vi "PID (Parallel) with monitoring.vi"(7 "Error":dbl, 12 "Proportional Gain":dbl=1.0, 13 "Integral Gain":dbl=1.0, 14 "Derivative Gain":dbl=1.0, 15 "High Frequency [s] (Tf)":dbl=1.0) -> (6 "Separate output":dbl[](array[numeric]), 8 "Output":dbl)   [LabVIEW 2017]
doc: "Constructs a PID model in transfer function form."
uses:
  <vilib>/Simulation/Model Libraries/PID/subVIs/SIM PID Derivative Gain.vi
  <vilib>/Simulation/Model Libraries/PID/subVIs/SIM PID Integral Gain.vi
  <vilib>/Simulation/Implementation/Shared/SIMSCR Execution Mode.ctl
  <vilib>/Simulation/Scripting/Companion Diagram/SimConfigNode/SimParams.ctl
  <vilib>/Simulation/Scripting/Companion Diagram/SimConfigNode/_simSolvers.ctl
  <vilib>/Simulation/Param Hierarchy/Typedefs/SIMPH Param Control Actions.ctl
  <vilib>/Simulation/Implementation/Shared/NILVSim_ParamChanged.vi
  <vilib>/Simulation/Implementation/Shared/NILVSIM_BeginStep.vi
  <vilib>/Simulation/SignalArithmetic/Implementation/NILVSim Gain.llb/SIM Gain (scalar).vi
  <vilib>/Simulation/Implementation/Shared/NILVSim_Manager.vi
  <vilib>/Utility/error.llb/Clear Errors.vi
  <vilib>/Simulation/Implementation/Shared/NILVSim_FinalizeModel.vi
  <vilib>/Simulation/Implementation/Shared/SIM Unbundle Sim Info.vi
  <vilib>/Simulation/Implementation/Shared/SIMSH Read Queue.vi
  <vilib>/Simulation/Implementation/Shared/NILVSim_Initialize.vi
  <vilib>/Simulation/Utility/Implementation/NILVSim Get Time and IsAcceptedStep.vi
  <vilib>/Simulation/Implementation/Shared/NILVSim_GetModelError.vi
  <vilib>/Simulation/Implementation/Shared/SIM SimErrorHandler.vi
  <vilib>/Simulation/Implementation/Shared/SIM Bundle Sim Info.vi
  <vilib>/Simulation/Scripting/Companion Diagram/SimConfigNode/SimDog.xnode
  <vilib>/Simulation/Implementation/XNodeFramework/SimXNode/SimX.xnode
  <vilib>/Simulation/Implementation/Shared/NI_SIM_Implementation.lvlib
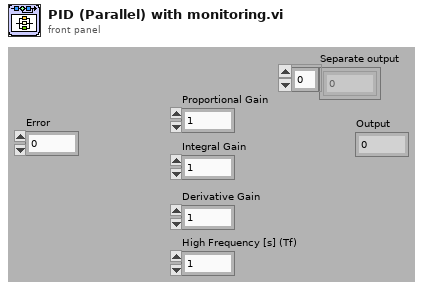
[diagram p1: front panel]
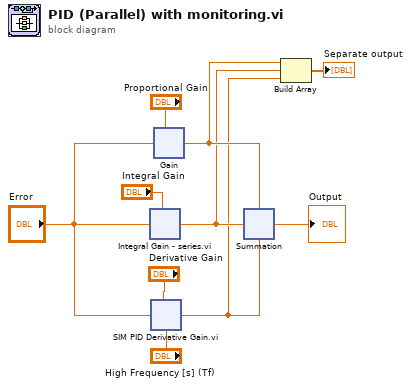
[diagram p0: block diagram]
diagram:
  n1 = xnode ("Integral Gain - series.vi")("Integral Gain"="Integral Gain", "Error"="Error") -> ("output"=w3:dbl)  [unwired: 2 in, 11 out]
  n2 = xnode ("SIM PID Derivative Gain.vi")("Derivative Gain"="Derivative Gain", "Error"="Error", "High Frequency [s] (Tf)"="High Frequency [s] (Tf)") -> ("output"=w2:dbl)  [unwired: 12 out]
  n3 = xnode ("Gain")("gain"="Proportional Gain", "input"="Error") -> ("output"=w4:dbl)  [unwired: 2 in]
  n4 = xnode ("Summation")("Operand1"=w4, "Operand2"=w3, "Operand3"=w2) -> ("Result"=→"Output":dbl)
  n5 = Build Array(w4, w3, w2) -> (→"Separate output":dbl[])
